vi "DAQmx Create Channel (AI-Bridge).vi"(0 "task in":refnum<k21>, 1 "maximum value":dbl=0.002 format="%.3f", 2 "minimum value":dbl=-0.002 format="%.3f", 3 "bridge information":T1={"bridge configuration"=10182, "voltage excitation source"=10200, "voltage excitation value"=2.5, "nominal bridge resistance"=350.0} {"voltage excitation source" items=["Internal"=10200, "External"=10167]; "bridge configuration" items=["Full Bridge"=10182, "Half Bridge"=10187, "Quarter Bridge"=10270]}, 5 "physical channels":tag, 7 "name to assign":string, 9 "units":i32(ring)=15896 items=["Volts/Volt"=15896, "mVolts/Volt"=15897, "From Custom Scale"=10065], 11 "error in":errorcluster, 12 "custom scale name":tag) -> (4 "task out":refnum<k21>, 15 "error out":errorcluster)   [LabVIEW 2013]
doc: "Creates channel(s) that measure voltage ratios from a Wheatstone bridge. Use this instance with bridge-based sensors that measure phenomena other than strain, force, pressure, or torque, or that scale data to physical units NI-DAQmx does not support."
uses:
  C:/Program Files (x86)/National Instruments/LabVIEW 2013/resource/objmgr/daqmx.rc
panel:
  # "input limits"
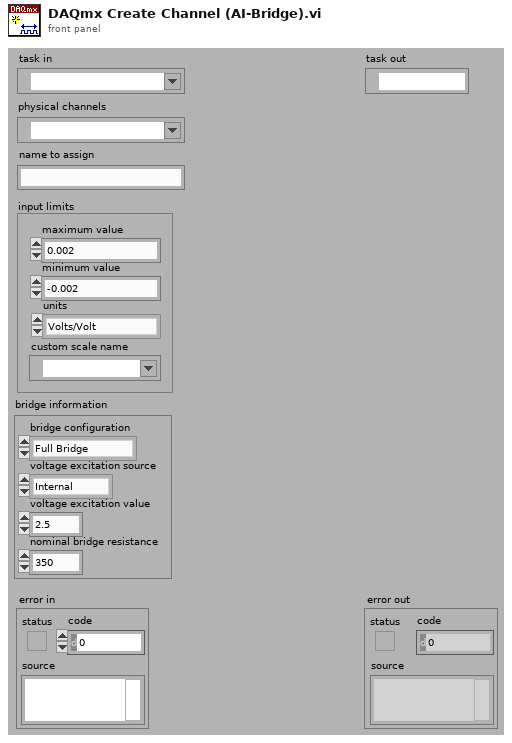
[diagram p1: front panel]
types:
  T1 = cluster{"bridge configuration":i32, "voltage excitation source":i32, "voltage excitation value":dbl, "nominal bridge resistance":dbl}
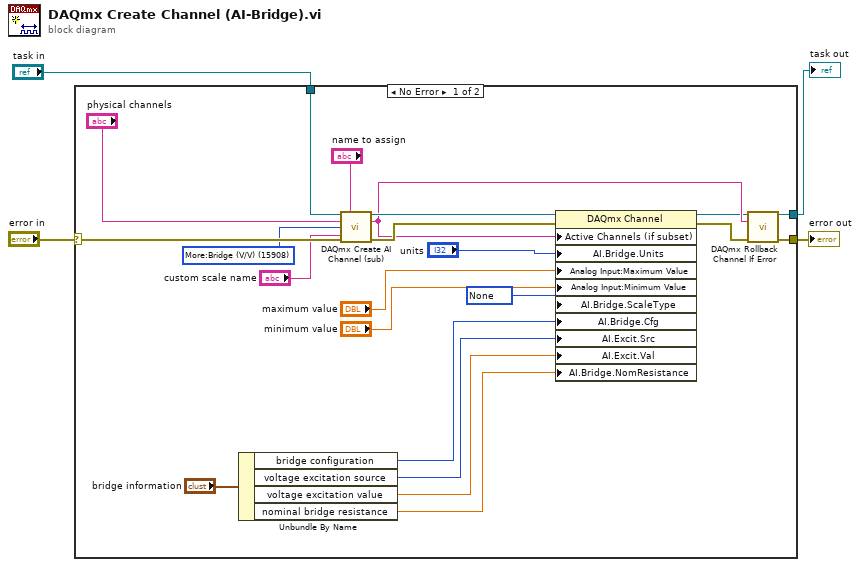
[diagram p0: block diagram]
diagram:
  n1 = case shown="No Error" "error in" {
    selector: "error in" -> [w25 w27]
    tunnel: [w17 w27] -> w4
    tunnel: "task in" -> [w26 w28]
    tunnel: [w16 w28] -> w1
    frame No Error {
      w6 = 10230 items=["None"=10230, "Two-Point Linear"=15898, "Table"=10450, "Polynomial"=10449] ("AI.Bridge.ScaleType")
      w12 = 15908 items=["Voltage"=10322, "Voltage RMS"=10350, "Current"=10134, "Current RMS"=10351, "More:Voltage:Custom with Excitation"=10323, "More:Bridge (V/V)"=15908, "Frequency"=10181, "Resistance"=10278, "Temperature:Thermocouple"=10303, "Temperature:Thermistor"=10302, "Temperature:RTD"=10301, "Temperature:Built-in Sensor"=10311, "Strain Gage"=10300, "Position:LVDT"=10352, "Position:RVDT"=10353, "Position:Eddy Current Proximity Probe"=14835, "Accelerometer"=10356, "Force:Bridge (Two-Point Linear)"=15899, "Force:Bridge (Table)"=15900, "Force:Bridge (Polynomial)"=15901, "Force:IEPE Sensor"=15895, "Pressure:Bridge (Two-Point Linear)"=15902, "Pressure:Bridge (Table)"=15903, "Pressure:Bridge (Polynomial)"=15904, "Sound Pressure:Microphone"=10354, "Torque:Bridge (Two-Point Linear)"=15905, "Torque:Bridge (Table)"=15906, "Torque:Bridge (Polynomial)"=15907, "TEDS Sensor"=12531] ("AI.MeasType")
      n2 = Unbundle By Name("bridge information") -> ("bridge configuration"=w10:i32, "voltage excitation source"=w9:i32, "voltage excitation value"=w8:dbl, "nominal bridge resistance"=w7:dbl)
      n3 = call "DAQmx Create AI Channel (sub).vi"("task in"=w26, "virtual channel name"="name to assign", "physical channel name"="physical channels", "measurement type"=w12, "error in"=w25, "custom scale"="custom scale name") -> ("task out"=w18:refnum<k21>, "channel names"=w15:string, "error out"=w23:errorcluster)  [unwired: 7 out]
      n4 = property class="DAQmx Channel"(reference=w18, error in=w23, "Active Channels (if subset)"=w15, "AI.Bridge.Units"="units", "Analog Input:Maximum Value"="maximum value", "Analog Input:Minimum Value"="minimum value", "AI.Bridge.ScaleType"=w6, "AI.Bridge.Cfg"=w10, "AI.Excit.Src"=w9, "AI.Excit.Val"=w8, "AI.Bridge.NomResistance"=w7) -> (reference out=w14:refnum<k21>, error out=w13:errorcluster)
      n5 = call "DAQmx Rollback Channel If Error.vi"("task in"=w14, "channel names"=w15, "error in"=w13) -> ("task out"=w16:refnum<k21>, "error out"=w17:errorcluster)  [unwired: 11 out]
    }
    frame Error {
    }
  }
  "error out" <- w4
  "task out" <- w1
